vi "Get Root Test.vi"(8 "error in (no error)":errorcluster, 9 "index (0: root)":i32, 11 "Test Event Storage in":refnum<class "Test Event Storage.lvclass">) -> (0 "error out":errorcluster, 2 "Test":string, 3 "Test Event Storage out":refnum<class "Test Event Storage.lvclass">)   [LabVIEW 2013, in "Caraya.lvlib" / "Test Event Storage.lvclass"]
uses:
  Test Event Storage.lvclass
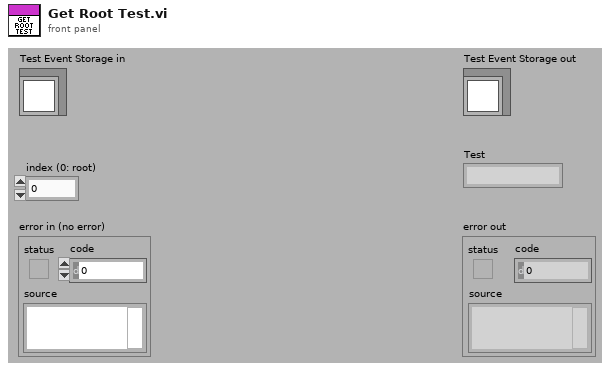
[diagram p1: front panel]
types:
  T1 = typedef "Caraya.lvlib/Test Result.lvclass/Assert Event Data.ctl" = cluster{"Name":string, "Passed":bool, "Call Chain":string[], "Test Error":errorcluster, "Time Stamp":timestamp, "Unique Assert ID":string, "Test ID":string, "Execution time (s)":dbl, "Verbose Explanation":string, "properties":variant, "measurements":variant, "limits":variant}
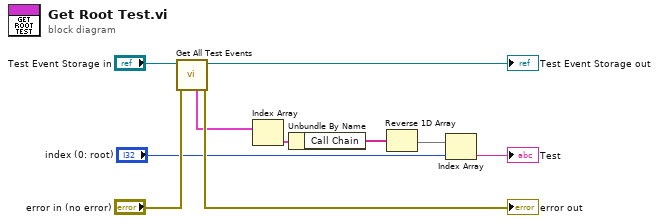
[diagram p0: block diagram]
diagram:
  n1 = call-dynamic "Get All Test Events.vi"("error in (no error)"="error in (no error)", "Test Event Storage in"="Test Event Storage in") -> ("error out"=→"error out":errorcluster, "Test Event Storage out"=→"Test Event Storage out":refnum<class "Test Event Storage.lvclass">, "Assertions"=w4:T1[])  [unwired: 6 in, 1 out]
  n2 = Index Array(array=w4) -> (element=w2:T1)  [unwired: 1 in]
  n3 = Unbundle By Name(w2) -> ("Call Chain"=w1:string[])
  n4 = Reverse 1D Array(array=w1) -> (reversed array=w3:string[])
  n5 = Index Array(array=w3, index="index (0: root)") -> (element=→"Test":string)
